vi "Check Multiplicity.vi"(10 "Residues":cdb[][](array[numeric]), 11 "Multiplicity In":i32[](array[numeric])) -> (0 "error":i32, 3 "Multiplicity Out":i32[](array[numeric]))   [LabVIEW 2014, in "NI_AALPro.lvlib"]
uses:
  NI_AALPro.lvlib
  Remove Zero Coefficients (CDB).vi
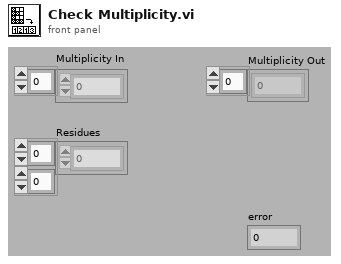
[diagram p1: front panel]
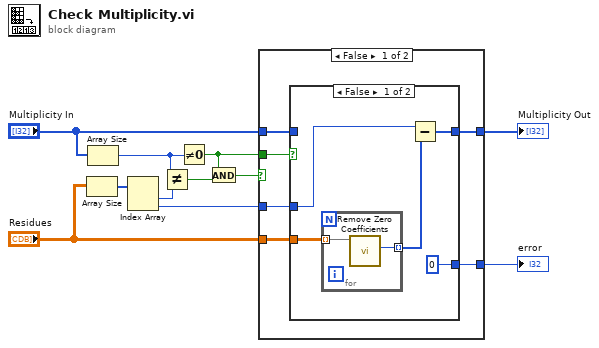
[diagram p0: block diagram]
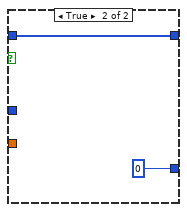
[diagram p2: hidden frame]
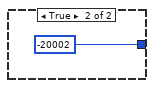
[diagram p3: hidden frame]
diagram:
  n1 = Array Size(array="Residues") -> (size(s)=w8:i32[])
  n2 = Array Size(array="Multiplicity In") -> (size(s)=w5:i32)
  n3 = Index Array(array=w8) -> (element #1=w6:i32, element #2=w1:i32)  [unwired: 2 in]
  n4 = Not Equal?(x=w5, y=w6) -> (x != y?=w3:bool)
  n5 = Not Equal To 0?(x=w5) -> (x != 0?=w2:bool)
  n6 = And(x=w2, y=w3) -> (x .and. y?=w4:bool)
  n7 = case shown="False" w4 {
    tunnel: [w17 _] -> w11
    tunnel: "Multiplicity In" -> [w16 _]
    tunnel: "Residues" -> [w15 _]
    tunnel: [w14 -20002] -> w7
    tunnel: w2 -> [w13 _]
    tunnel: w1 -> [w12 _]
    frame False {
      n8 = case shown="False" w13 {
        tunnel: w16 -> [_ w26]
        tunnel: w15 -> [w22 _]
        tunnel: [w18 w26] -> w17
        tunnel: [0 0] -> w14
        tunnel: w12 -> [w20 _]
        frame False {
          n9 = for {
            tunnel: w22 -> [w24] mode=indexing
            tunnel: [w23] -> w19 mode=indexing
            n10 = call-poly "Remove Zero Coefficients.vi"("P(x) In"=w24) -> ("number of zero coefficients"=w23:i32)  [unwired: 8 in, 2 out]
          }
          n11 = Subtract(x=w20, y=w19) -> (x-y=w18:i32[])
        }
        frame True {
        }
      }
    }
    frame True {
    }
  }
  "Multiplicity Out" <- w11
  "error" <- w7
